vi "Write ITX (XY2).vi"(4 "Commands":string, 6 "Notes":string, 8 "error in":errorcluster, 9 "Wavenames":string[](array[string]), 10 "array of clusters":cluster{"Y  Array":dbl[]}[](array[cluster]), 11 "filename":path) -> (0 "error out":errorcluster, 3 "file":path)   [LabVIEW 2020, in "Data.ITX.lvclass"]
uses:
  Data.ITX.lvclass
panel:
  out "String":string
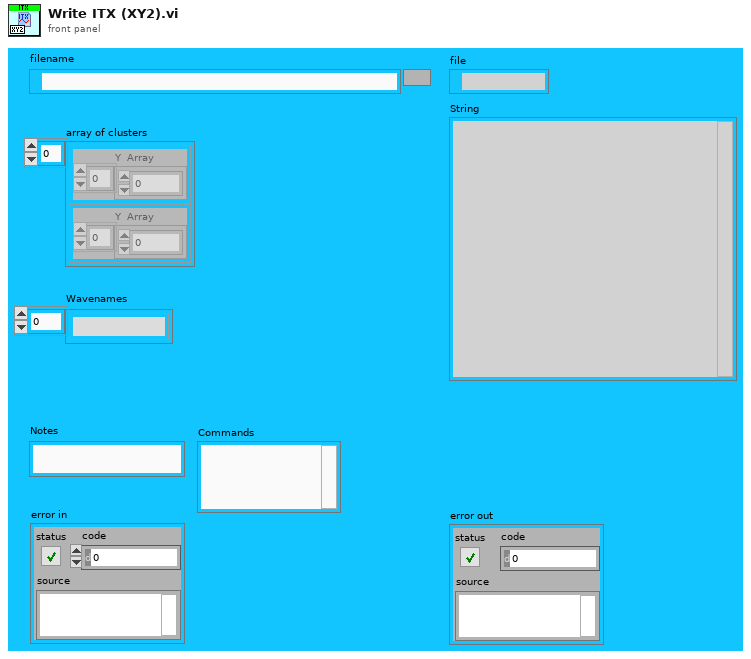
[diagram p1: front panel]
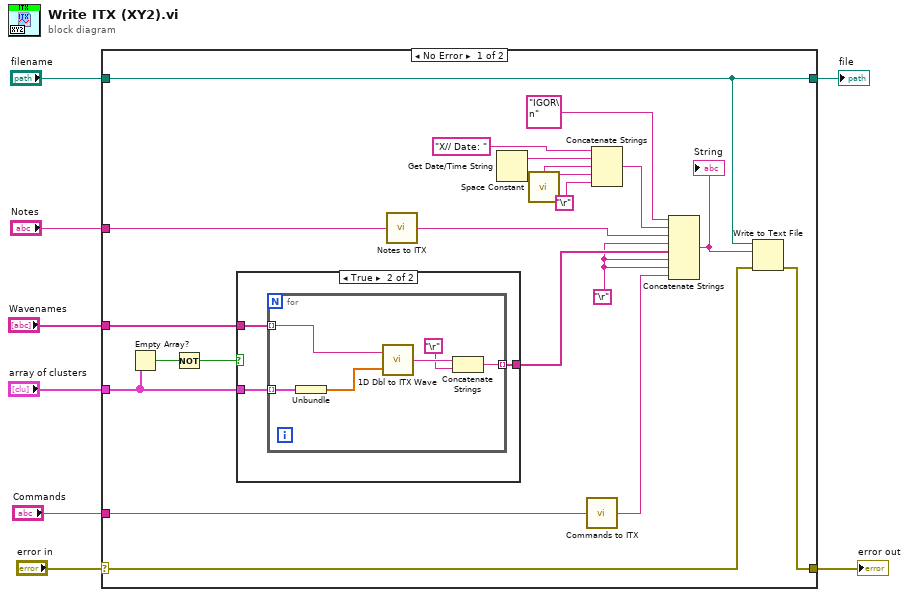
[diagram p0: block diagram]
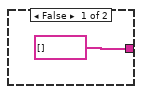
[diagram p2: hidden frame]
diagram:
  n1 = case shown="No Error" "error in" {
    selector: "error in" -> [w14 w41]
    tunnel: "Notes" -> [w22 _]
    tunnel: "array of clusters" -> [w12 _]
    tunnel: "filename" -> [w15 w40]
    tunnel: [w17 w41] -> w5
    tunnel: [w15 w40] -> w4
    tunnel: "Wavenames" -> [w11 _]
    tunnel: "Commands" -> [w10 _]
    frame No Error {
      w9 = "\r"
      n2 = Empty Array?(array=w12) -> (empty?=w23:bool)
      n3 = Not(x=w23) -> (.not. x?=w16:bool)
      n4 = case shown="True" w16 {
        tunnel: w12 -> [_ w33]
        tunnel: [string[] [] w32] -> w13
        tunnel: w11 -> [_ w31]
        frame False {
        }
        frame True {
          n5 = for {
            tunnel: [w39] -> w32 mode=indexing
            tunnel: w33 -> [w36] mode=indexing
            tunnel: w31 -> [w34] mode=indexing
            n6 = Unbundle(w36) -> ("Y  Array"=w35:dbl[])
            n7 = call "1D Dbl to ITX Wave.vi"("1D Array"=w35, "Wavename"=w34) -> ("ITX Wave"=w38:string)
            n8 = Concatenate Strings(w38, "\r") -> (w39:string)
          }
        }
      }
      n9 = call "Notes to ITX.vi"("Notes"=w22) -> ("ITX Notes"=w19:string)
      n10 = Get Date/Time String() -> (date string=w28:string, time string=w29:string)  [unwired: 3 out]
      n11 = call <vilib>:"Space Constant.vi"() -> ("String"=w26:string)
      n12 = call "Commands to ITX.vi"("Commands"=w10) -> ("ITX Commands"=w18:string)
      n13 = Concatenate Strings("X// Date: " ("format string"), w28, w26, w29, "\r") -> (w21:string)
      n14 = Concatenate Strings("IGOR\n", w21, w19, w9, w13, w9, w9, w18) -> (w24:string)
      "String" <- w24
      n15 = Write to Text File(file (use dialog)=w15, text=w24, error in=w14) -> (error out=w17:errorcluster)  [unwired: 3 out]
    }
    frame Error {
    }
  }
  "file" <- w4
  "error out" <- w5
